vi "ASCII Command-Response.vi"() -> ()   [LabVIEW 2019]
uses:
  <vilib>/Instr/_visa.llb/VISA Configure Serial Port (Instr).vi
panel:
  in  "Send":bool
  in  "Command":string(combo)
  out "read buffer":string
  out "error out":errorcluster
  in  "VISA resource name":refnum<visa-resource-name>
  # "To test this code, use a NULL Modem cable and use ASCII Intermittent.vi to act as the instrument"
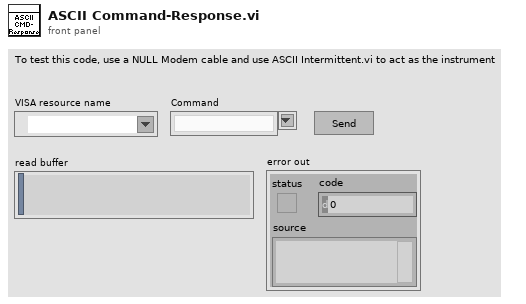
[diagram p1: front panel]
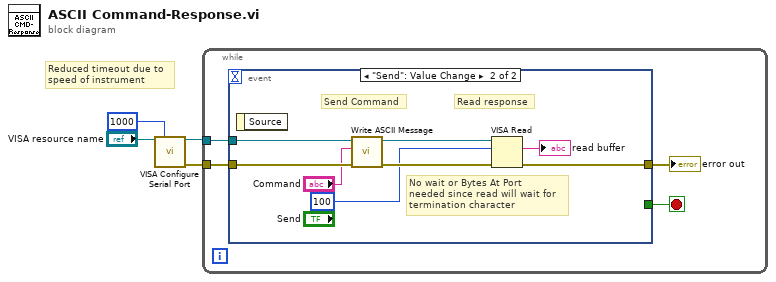
[diagram p0: block diagram]
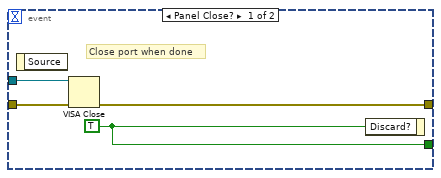
[diagram p2: hidden frame]
diagram:
  # "Reduced timeout due to\nspeed of instrument"
  n1 = call-poly "VISA Configure Serial Port"("VISA resource name"="VISA resource name", "timeout (10sec)"=u32 1000) -> ("VISA resource name out"=w2:refnum<visa-resource-name>, "error out"=w4:errorcluster)  [unwired: 12 in]
  n2 = while {
    tunnel: w4 -> [w8]
    tunnel: w2 -> [w6]
    stop <- w5 stop-if-true
    n3 = event shown="[1] \"Send\": Value Change" {
      selector: _ -> [_ _]
      dyn-events: _ -> [_ _]
      timeout: _ -> [_ _]
      tunnel: w8 -> [w12 w20]
      tunnel: w6 -> [w10 w17]
      tunnel: [w11 w18] -> w7
      tunnel: [w9 _] -> w5
      event Panel Close? {
        w9 = TRUE ("stop")
        # "Close port when done"
        n4 = event-data() -> ()  [unwired: 1 in, 1 out]
        n5 = VISA Close(VISA resource name=w10, error in (no error)=w12) -> (error out=w11:errorcluster)
        n6 = event-data("Discard?"=w9) -> ()  [unwired: 1 in, 1 out]
      }
      event "Send": Value Change {
        # "No wait or Bytes At Port\nneeded since read will wait for\ntermination character"
        # "Read response"
        # "Send Command"
        n7 = event-data() -> ()  [unwired: 1 in, 1 out]
        n8 = call "Write ASCII Message.vi"("error in"=w20, "Message"="Command", "VISA resource in"=w17) -> ("error out"=w19:errorcluster, "VISA resource out"=w15:refnum<visa-resource-name>)  [unwired: 7 in]
        n9 = VISA Read(VISA resource name=w15, byte count=u32 100, error in (no error)=w19) -> (read buffer=→"read buffer":string, error out=w18:errorcluster)  [unwired: 2 out]
      }
    }
    "error out" <- w7
  }
